vi "Present Data.vi"(8 "error in (no error)":errorcluster, 10 "Debug Data":refnum<class "Debug Data.lvclass">[](array[class]), 11 "List Box View Model In":refnum<class "List Box Event Log View Model.lvclass">) -> (0 "error out":errorcluster, 2 "Data Out":string[][](array[string]), 3 "List Box View Model Out":refnum<class "List Box Event Log View Model.lvclass">)   [LabVIEW 2020, in "List Box Event Log View Model.lvclass"]
uses:
  List Box Event Log View Model.lvclass
  Debug Data/Debug Data.lvclass
  Debug Data/Debug Data.lvclass/Debug Data.ctl
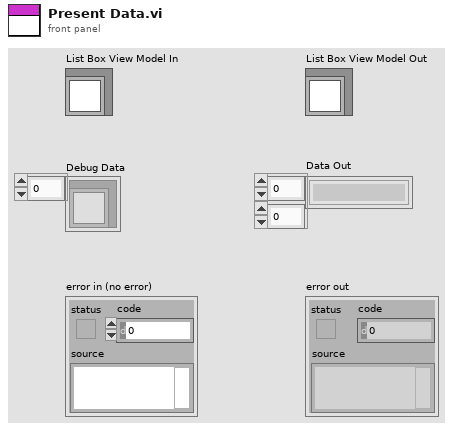
[diagram p1: front panel]
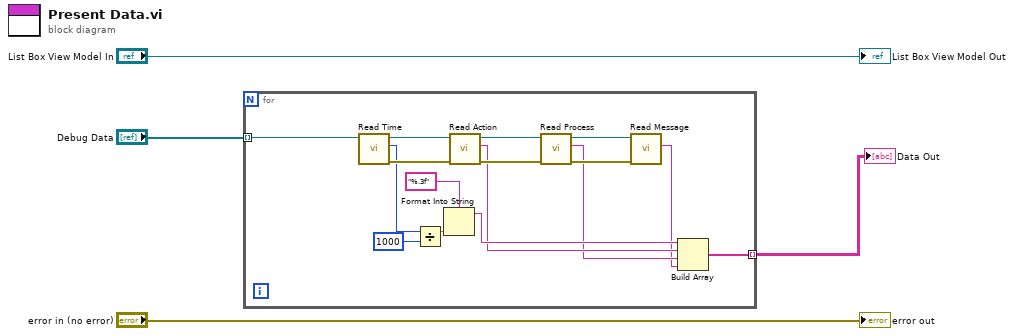
[diagram p0: block diagram]
diagram:
  n1 = for {
    tunnel: "Debug Data" -> [w17] mode=indexing
    tunnel: [w5] -> w1 mode=indexing
    n2 = call "Read Time.vi"("Debug Data in"=w17) -> ("error out"=w20:errorcluster, "Time"=w16:u32, "Debug Data out"=w10:refnum<class "Debug Data.lvclass">)  [unwired: 8 in]
    n3 = Divide(x=w16, y=u32 1000) -> (x/y=w15:dbl)
    n4 = Format Into String(format string="%.3f", w15) -> (resulting string=w12:string)  [unwired: 2 in, 1 out]
    n5 = call "Read Action.vi"("error in (no error)"=w20, "Debug Data in"=w10) -> ("error out"=w11:errorcluster, "Action"=w8:string, "Debug Data out"=w9:refnum<class "Debug Data.lvclass">)  [unwired: 7 in]
    n6 = call "Read Process.vi"("error in (no error)"=w11, "Debug Data In"=w9) -> ("error out"=w18:errorcluster, "Process"=w7:string, "Debug Data Out"=w19:refnum<class "Debug Data.lvclass">)  [unwired: 7 in]
    n7 = call "Read Message.vi"("error in (no error)"=w18, "Debug Data in"=w19) -> ("Message"=w6:string)  [unwired: 6 in, 3 out]
    n8 = Build Array(w12, w8, w7, w6) -> (w5:string[])
  }
  "Data Out" <- w1
  "error out" <- "error in (no error)"
  "List Box View Model Out" <- "List Box View Model In"
